vi "Resample Time Series.vi"() -> ()   [LabVIEW 2023]
doc: "This example shows how to resample a univariate time series with the TSA Resampling VI.\n\n<b>Instructions:</b>\n1) Run this VI.\n2) Set the new sampling rate.\n3) Stop this VI.\n4) Zoom in the plot to observe the resampled signal against the original signal."
uses:
  <vilib>/addons/Time Series Analysis/Utilities.llb/TSA Data.ctl
  <vilib>/addons/Time Series Analysis/Series Preprocess.llb/TSA Resampling (Waveform).vi
  <vilib>/addons/_Advanced Signal Processing/NI_AdvSigProcTSA.lvlib
panel:
  in  "stop":bool
  out "Original sampling rate":dbl=1.0
  in  "New sampling rate":dbl=0.1
  out "Time Series":waveform(dbl)[](graph)
  # "Overview: Shows how to resample a univariate time series with the TSA Resampling VI.\nRequirements: LabVIEW Full Development System, Advanced Signal Processing Toolkit\nInstructions: \n1. Run this VI.\n2. Set the new sampling rate.\n3. Stop this VI.\n4. Zoom in the plot to observe the resampled signal against the original signal.\n5.  Click Stop to stop the VI."
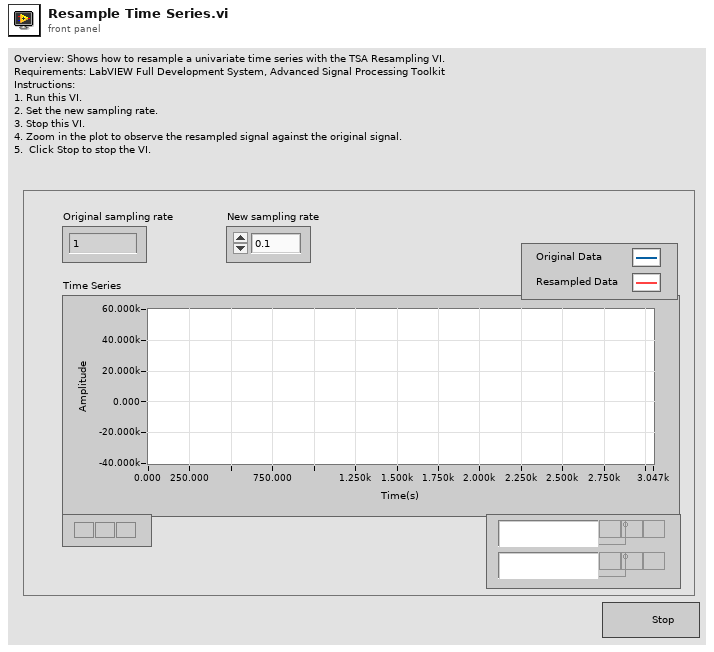
[diagram p1: front panel]
types:
  T1 = typedef "NI_AdvSigProcTSA.lvlib/TSA Data.ctl" = u16
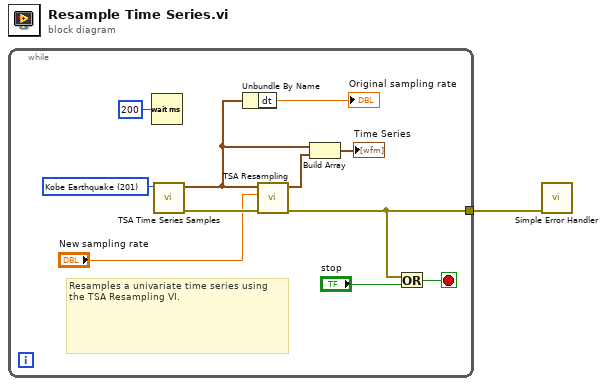
[diagram p0: block diagram]
diagram:
  n1 = while {
    tunnel: [w2] -> w1
    stop <- w5 stop-if-true
    w3 = T1 201 items=["Kobe Earthquake"=201, "EEG"=210, "Bearing Vibration (simulated)"=211, "Period Product Sales"=214, "Beam Vibration (nonlinear)"=217, "Beam Vibration (linear)"=218, "Signal With Echo"=219, "Engine Knocking"=220, "Power Line"=221, "-"=200, "Beam Deflections (multivariate)"=207, "Structure Vibration (multivariate)"=208, "Human MEG (multivariate)"=222] ("data")
    # "Resamples a univariate time series using the TSA Resampling VI."
    n2 = Wait (ms)(milliseconds to wait=u32 200 ("millisecond multiple")) -> ()  [unwired: 1 out]
    n3 = call <vilib>:"TSA Time Series Samples.vi"("data"=w3) -> ("error out"=w12:errorcluster, "univariate time series"=w8:waveform(dbl))  [unwired: 1 in, 8 out]
    n4 = Unbundle By Name(w8) -> ("dt"=→"Original sampling rate":dbl)
    n5 = call-poly <vilib>:"TSA Resampling.vi"("error in (no error)"=w12, "new sampling rate"="New sampling rate", "Xt"=w8) -> ("error out"=w2:errorcluster, "Xt resampled"=w9:waveform(dbl))  [unwired: 7 out]
    n6 = Build Array(w8, w9) -> (→"Time Series":waveform(dbl)[])
    n7 = Or(x=w2, y="stop") -> (x .or. y?=w5:bool)
  }
  n8 = call <vilib>:"Simple Error Handler.vi"("error in (no error)"=w1) -> ()  [unwired: 1 in, 8 out]
